vi "ImageReader.vi"() -> ()   [LabVIEW 2013]
uses:
  ROS/Code/Functions.ctl
panel:
  in  "Functions":T1=[0, 2, 4]
  in  "stop":bool
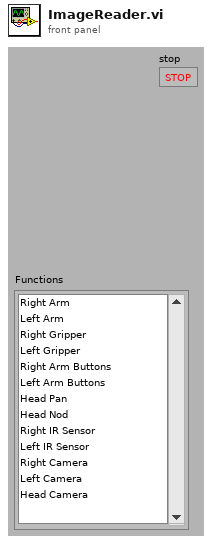
[diagram p1: front panel]
types:
  T1 = typedef "Functions.ctl" = i32[]
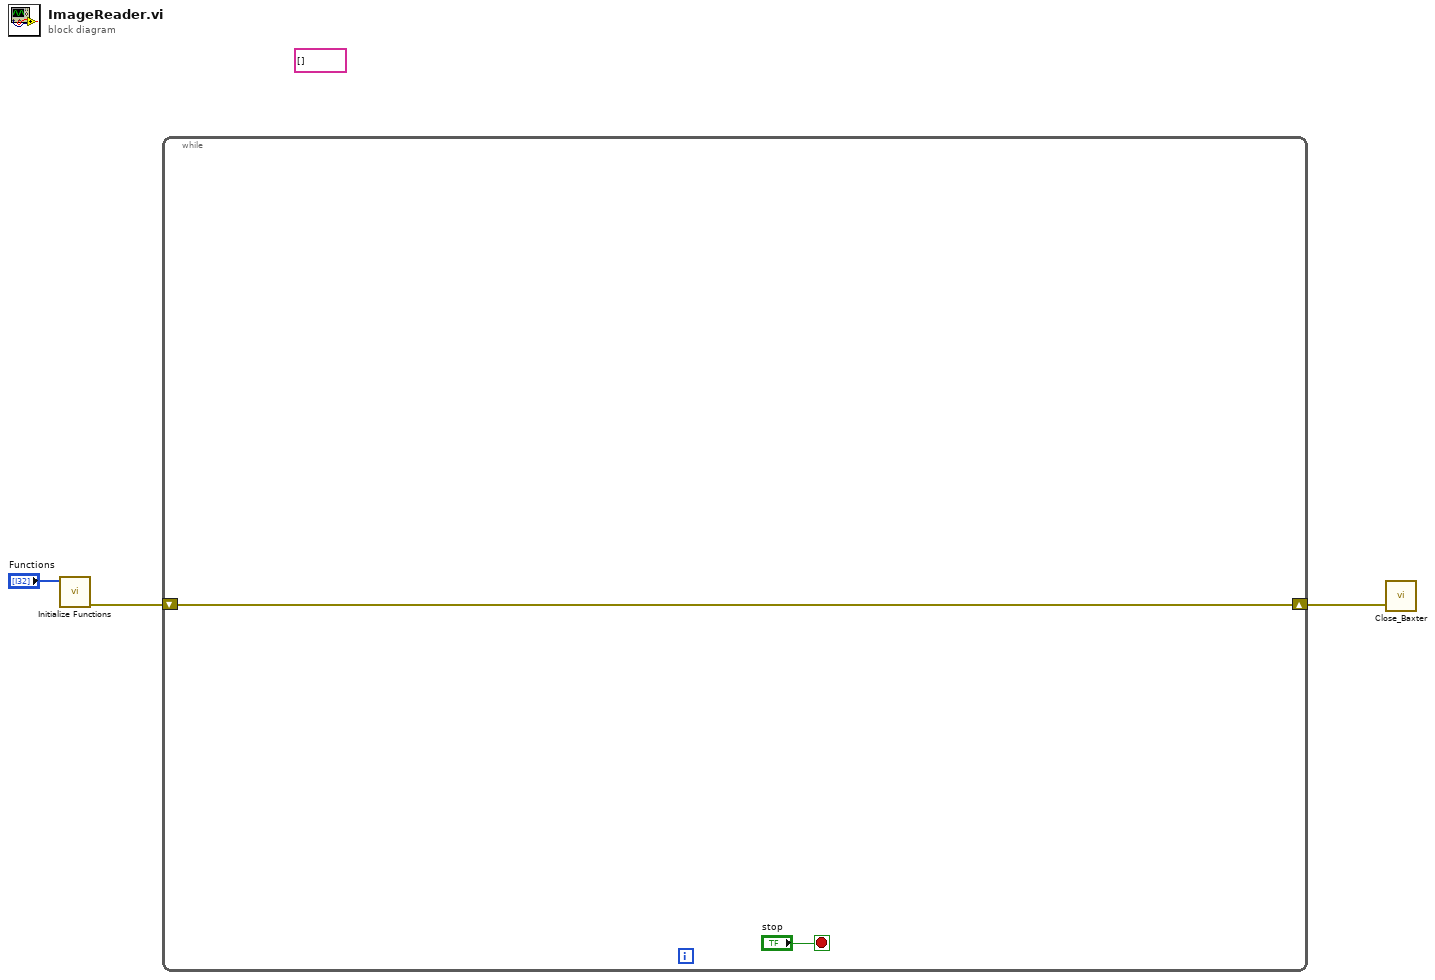
[diagram p0: block diagram]
diagram:
  (unwired) string[] [] ("Item Names")
  n1 = call "Initialize Functions.vi"("Functions"="Functions") -> ("error out"=w3:errorcluster)  [unwired: 10 in]
  n2 = while {
    shift-right: [w4] -> w2
    shift-left: w3 -> [w4]
    stop <- "stop" stop-if-true
  }
  n3 = call "Close_Baxter.vi"("error in"=w2) -> ()  [unwired: 3 in, 1 out]
